vi "Get Server DLL Path.vi"() -> (0 "Server dll path":path)   [LabVIEW 2016, in "Query Server.lvlib" / "gprc-lvsupport.lvlib"]
uses:
  gprc-lvsupport.lvlib
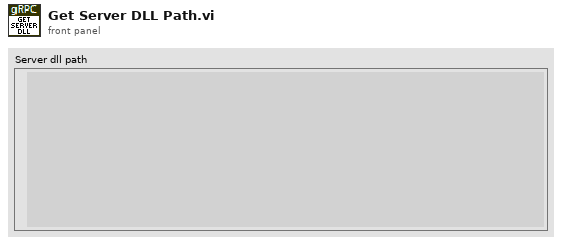
[diagram p1: front panel]
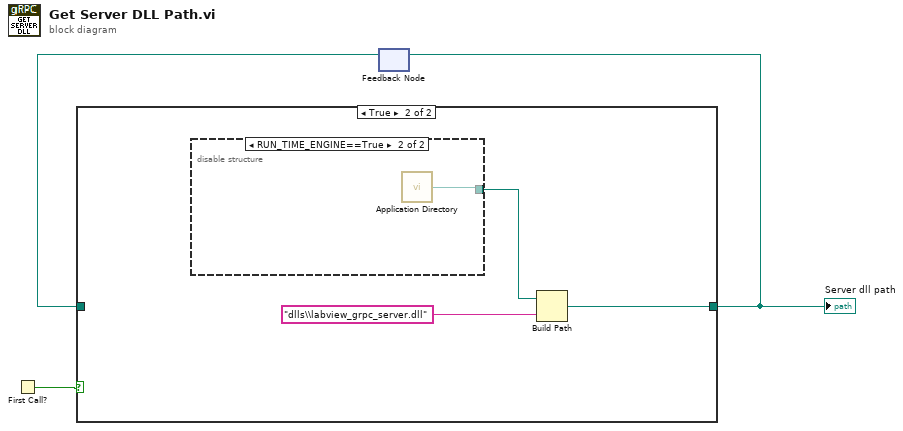
[diagram p0: block diagram]
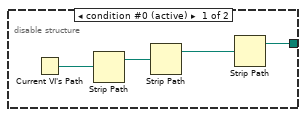
[diagram p3: hidden frame]
diagram:
  n1 = First Call?() -> (First Call?: T/F=w3:bool)
  n2 = feedback #1() -> (w1:path)  [unwired: 1 in]
  n3 = case shown="True" w3 {
    tunnel: [w4 w7] -> w2
    tunnel: w1 -> [w4 _]
    frame False {
    }
    frame True {
      n4 = disable-structure shown="RUN_TIME_ENGINE==True" {
        disable-tunnel: [w8 w12] -> w5
        frame condition #0 (active) {
          n5 = Current VI's Path() -> (path=w10:path)
          n6 = Strip Path(path=w10) -> (stripped path=w11:path)  [unwired: 1 out]
          n7 = Strip Path(path=w11) -> (stripped path=w9:path)  [unwired: 1 out]
          n8 = Strip Path(path=w9) -> (stripped path=w8:path)  [unwired: 1 out]
        }
        frame condition #1 {
          n9 = call <vilib>:"Application Directory.vi"() -> ("Application Directory"=w12:path)
        }
      }
      n10 = Build Path(base path=w5, name or relative path="dlls\\labview_grpc_server.dll") -> (appended path=w7:path)
    }
  }
  "Server dll path" <- w2
  n11 = feedback-in #1(w2) -> ()
